vi "LINE_v3s.vi"() -> ()   [LabVIEW 2010]
uses:
  <vilib>/express/express arith-compare/Formula/XNode/ExpressFormulaBlockNode.xnode
panel:
  in  "x-dist":i32
  in  "Motor GPIB":u8=6
  in  "speed":u16
  in  "y-dist":i32
  in  "Current (mA)":dbl
  in  "Laser GPIB":u8=10 max=100
  out "Dummy":string
  # "LINE<space>[Displacement]<space>[Speed]<space>[Current]"
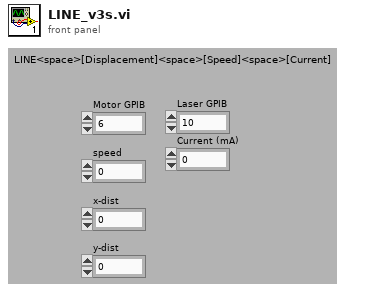
[diagram p1: front panel]
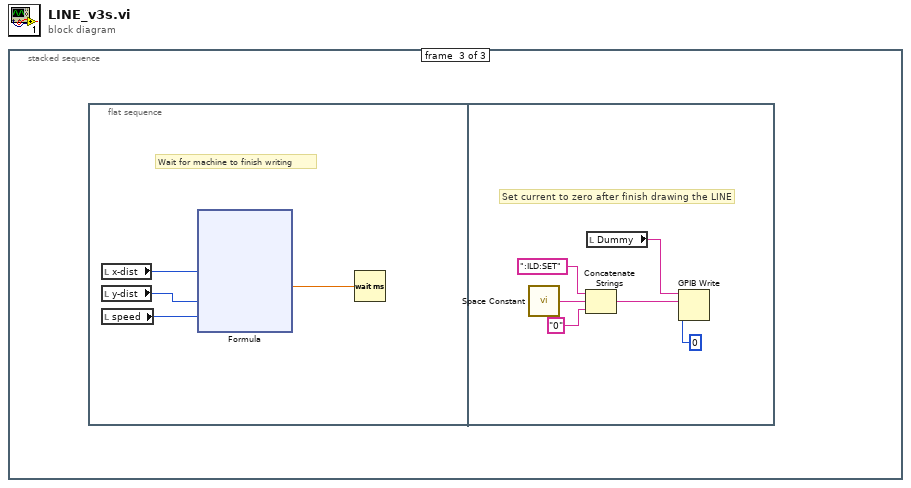
[diagram p0: block diagram]
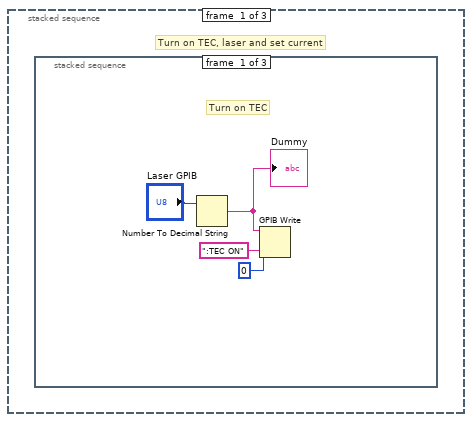
[diagram p2: hidden frame]
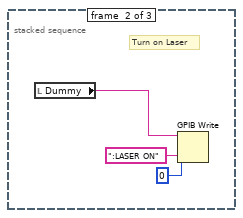
[diagram p3: hidden frame]
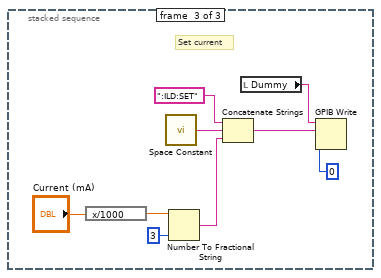
[diagram p4: hidden frame]
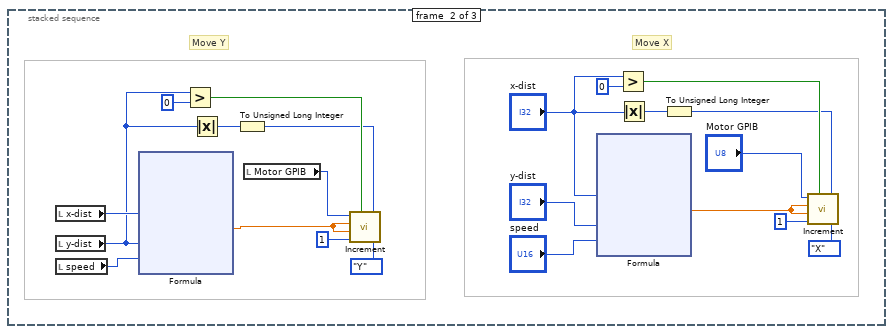
[diagram p5: hidden frame]
diagram:
  n1 = stacked-sequence {
    frame #0 {
      # "Turn on TEC, laser and set current"
      n2 = stacked-sequence {
        frame #0 {
          # "Turn on TEC"
          n3 = Number To Decimal String(number="Laser GPIB") -> (decimal integer string=w1:string)  [unwired: 1 in]
          "Dummy" <- w1
          n4 = GPIB Write(0:w1, 1:":TEC ON" ("data"), 2:i16 0 ("mode (0)")) -> ()  [unwired: 2 in, 2 out]
        }
        frame #1 {
          # "Turn on Laser"
          n5 = local read "Dummy"() -> (w5:string)
          n6 = GPIB Write(0:w5, 1:":LASER ON" ("data"), 2:i16 0 ("mode (0)")) -> ()  [unwired: 2 in, 2 out]
        }
        frame #2 {
          # "Set current"
          n7 = expression code="x/1000"("Current (mA)") -> (w12:dbl)
          n8 = call <vilib>:"Space Constant.vi"() -> ("String"=w14:string)
          n9 = Number To Fractional String(number=w12, precision (6)=i16 3) -> (F-format string=w9:string)  [unwired: 2 in]
          n10 = Concatenate Strings(":ILD:SET", w14, w9) -> (w13:string)
          n11 = local read "Dummy"() -> (w8:string)
          n12 = GPIB Write(0:w8, 1:w13, 2:i16 0 ("mode (0)")) -> ()  [unwired: 2 in, 2 out]
        }
      }
    }
    frame #1 {
      # "Move X"
      # "Move Y"
      n13 = local read "x-dist"() -> (w32:i32)
      n14 = local read "y-dist"() -> (w29:i32)
      n15 = local read "speed"() -> (w36:u16)
      n16 = xnode "Formula"("X1"=w32, "X2"=w29, "X3"=w36) -> ("Result"=w31:dbl)  [unwired: 1 in, 1 out]
      n17 = Greater?(x=w29, y=0) -> (0:w33:bool)
      n18 = Absolute Value(x=w29) -> (abs(x)=w30:i32)
      n19 = To Unsigned Long Integer(number=w30) -> (unsigned 32bit integer=w28:u32)
      n20 = local read "Motor GPIB"() -> (w35:u8)
      n21 = call "Increment.vi"("GPIB_Addr"=w35, "F Speed"=w31, "L Speed"=w31, "Rate"=u16 1, "CCW 3"=w33, "Distance"=w28, "Axis"=enum16{"X", "Y", "Z", "U", "V", "W"}."Y") -> ()
      n22 = xnode "Formula"("X1"="x-dist", "X2"="y-dist", "X3"="speed") -> ("Result"=w23:dbl)  [unwired: 1 in, 1 out]
      n23 = Greater?(x="x-dist", y=0) -> (0:w21:bool)
      n24 = Absolute Value(x="x-dist") -> (abs(x)=w18:i32)
      n25 = To Unsigned Long Integer(number=w18) -> (unsigned 32bit integer=w17:u32)
      n26 = call "Increment.vi"("GPIB_Addr"="Motor GPIB", "F Speed"=w23, "L Speed"=w23, "Rate"=u16 1, "CCW 3"=w21, "Distance"=w17, "Axis"=enum16{"X", "Y", "Z", "U", "V", "W"}."X") -> ()
    }
    frame #2 {
      n27 = flat-sequence {
        frame #0 {
          # "Wait for machine to finish writing"
          n28 = local read "x-dist"() -> (w66:i32)
          n29 = local read "y-dist"() -> (w65:i32)
          n30 = local read "speed"() -> (w64:u16)
          n31 = xnode "Formula"("X1"=w66, "X2"=w65, "X3"=w64) -> ("Result"=w63:dbl)  [unwired: 1 in, 1 out]
          n32 = Wait (ms)(milliseconds to wait=w63) -> ()  [unwired: 1 out]
        }
        frame #1 {
          # "Set current to zero after finish drawing the LINE"
          n33 = call <vilib>:"Space Constant.vi"() -> ("String"=w82:string)
          n34 = Concatenate Strings(":ILD:SET", w82, "0" ("string")) -> (w81:string)
          n35 = local read "Dummy"() -> (w79:string)
          n36 = GPIB Write(0:w79, 1:w81, 2:i16 0 ("mode (0)")) -> ()  [unwired: 2 in, 2 out]
        }
      }
    }
  }
